vi "Write FIFOs.vi"(7 "Mode":T1, 8 "error in (no error)":errorcluster, 11 "RT Data in":T2 {"Label Transfer Config"."Block Data Refs"."Data Reference" format="%.0x"; "Status Config"."HWOut Dur Ref" format="%.0x"; "Status Config"."HWIn Dur Ref" format="%.0x"; "Status Config"."Error Data Ref" format="%.0x"; "HWOutput Channels"."Labels Settings"."Label" format="%.0o"; "HWInput Channels"."Labels Settings"."Label" format="%.0o"}) -> (0 "error out":errorcluster, 3 "RT Data out":T2 {"Label Transfer Config"."Block Data Refs"."Data Reference" format="%.0x"; "Status Config"."HWOut Dur Ref" format="%.0x"; "Status Config"."HWIn Dur Ref" format="%.0x"; "Status Config"."Error Data Ref" format="%.0x"; "HWOutput Channels"."Labels Settings"."Label" format="%.0o"; "HWInput Channels"."Labels Settings"."Label" format="%.0o"})   [LabVIEW 2017]
uses:
  RT Controls/RT Data.ctl
  RT Controls/RT HW Channel.ctl
  RT Controls/RT Label Settings.ctl
  Shared/Controls and Global/Label.ctl
  Shared/Controls and Global/transferPeriod.ctl
  RT Controls/Driver Data.ctl
  RT Controls/RT Word Settings.ctl
  <vilib>/NI Veristand/Custom Device API/Block Data Reference.ctl
  <vilib>/NI Veristand/Custom Device API/Data Reference.ctl
  RT Controls/RT Param Setting.ctl
  Shared/Controls and Global/Start Bit.ctl
  Shared/Controls and Global/Number of Bits.ctl
  Shared/Controls and Global/TransferType.ctl
  RT Controls/Error Qs.ctl
  RT Controls/Status Channels Config.ctl
  RT Controls/FIFO.ctl
  RT Controls/Label Transfer Config.ctl
  RT Controls/ReadWrite Selector.ctl
  Shared/Ballard Arinc-429 Shared.lvlib
  <vilib>/NI Veristand/Custom Device API/Custom Device API.lvlib
  Ballard Arinc-429 Engine.lvlib
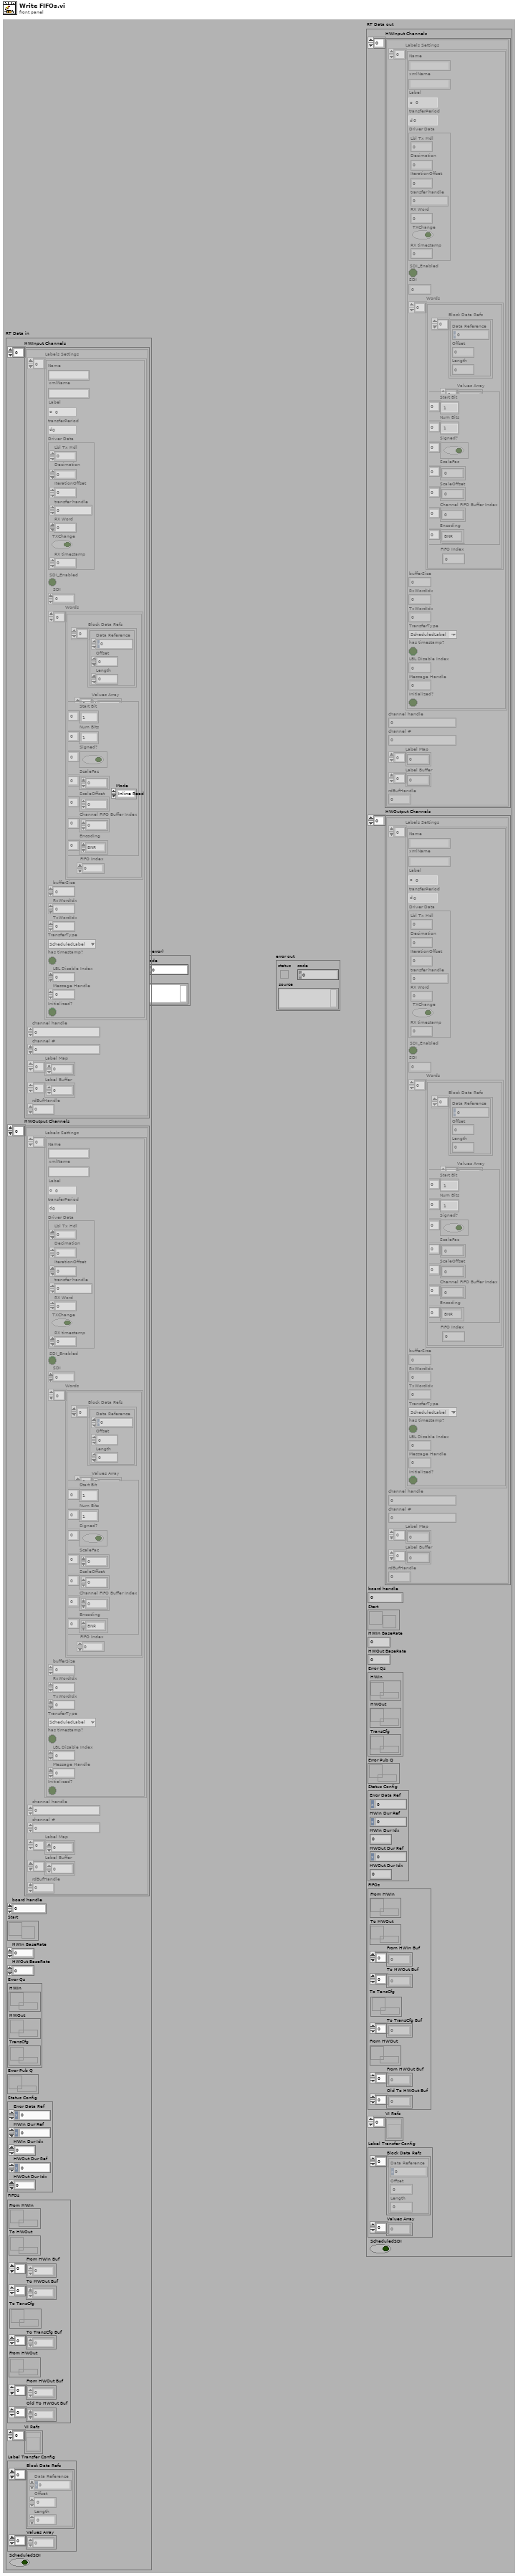
[diagram p1: front panel]
types:
  T1 = typedef "Ballard Arinc-429 Engine.lvlib/ReadWrite Selector.ctl" = enum16{"Inline Read", "Inline Write", "Async HWIn", "Async HWOut"}
  T2 = typedef "Ballard Arinc-429 Engine.lvlib/RT Data.ctl" = cluster{"HWInput Channels":T3[], "HWOutput Channels":T3[], "board handle":u32, "Start":refnum<notifier>, "HWIn BaseRate":i64, "HWOut BaseRate":i64, "Error Qs":T15, "Error Pub Q":refnum<queue>, "Status Config":T16, "FIFOs":T17, "VI Refs":refnum<vi>[], "Label Transfer Config":T18, "ScheduledSDI":bool}
  T3 = typedef "Ballard Arinc-429 Engine.lvlib/RT HW Channel.ctl" = cluster{"Labels Settings":T4[], "channel handle":u32, "channel #":u16, "Label Map":i32[], "Label Buffer":u32[], "rdBufHandle":u32}
  T4 = typedef "Ballard Arinc-429 Engine.lvlib/RT Label Settings.ctl" = cluster{"Name":string, "xmlName":string, "Label":T5, "transferPeriod":T6, "Driver Data":T7, "SDI_Enabled":bool, "SDI":u8, "Words":T8[], "bufferSize":u32, "RxWordIdx":i32, "TxWordIdx":i32, "TransferType":T14, "has timestamp?":bool, "LBL Disable Index":i32, "Message Handle":u64, "Initialized?":bool}
  T5 = typedef "Ballard Arinc-429 Shared.lvlib/Label.ctl" = u8
  T6 = typedef "Ballard Arinc-429 Shared.lvlib/transferPeriod.ctl" = u32
  T7 = typedef "Driver Data.ctl" = cluster{"Lbl Tx Hdl":u32, "Decimation":i32, "IterationOffset":i32, "transfer handle":u32, "RX Word":u32, "TXChange":bool, "RX timestamp":dbl}
  T8 = typedef "Ballard Arinc-429 Engine.lvlib/RT Word Settings.ctl" = cluster{"Block Data Refs":T9[], "Values Array":dbl[], "Length":i32, "FIFO Index":i32, "Param Setting":T11}
  T9 = typedef "Custom Device API.lvlib/Block Data Reference.ctl" = cluster{"Data Reference":T10, "Offset":u64, "Length":u64}
  T10 = typedef "Custom Device API.lvlib/Data Reference.ctl" = i32
  T11 = typedef "Ballard Arinc-429 Engine.lvlib/RT Param Setting.ctl" = cluster{"Start Bit":T12[], "Num Bits":T13[], "Signed?":bool[], "ScaleFac":dbl[], "ScaleOffset":dbl[], "Channel FIFO Buffer Index":i32[], "Encoding":enum16{"BNR", "BCD", "Discrete"}[]}
  T12 = typedef "Ballard Arinc-429 Shared.lvlib/Start Bit.ctl" = i32
  T13 = typedef "Ballard Arinc-429 Shared.lvlib/Number of Bits.ctl" = i32
  T14 = typedef "Ballard Arinc-429 Shared.lvlib/TransferType.ctl" = enum16{"ScheduledLabel", "Acyclic", "Block", "Strobe"}
  T15 = typedef "Error Qs.ctl" = cluster{"HWIn":refnum<queue>, "HWOut":refnum<queue>, "TransCfg":refnum<queue>}
  T16 = typedef "Ballard Arinc-429 Engine.lvlib/Status Channels Config.ctl" = cluster{"Error Data Ref":T10, "HWIn Dur Ref":T10, "HWIn Dur Idx":i32, "HWOut Dur Ref":T10, "HWOut Dur Idx":i32}
  T17 = typedef "FIFO.ctl" = cluster{"From HWIn":refnum<k33>, "To HWOut":refnum<k33>, "From HWIn Buf":dbl[], "To HWOut Buf":dbl[], "To TansCfg":refnum<k33>, "To TransCfg Buf":dbl[], "From HWOut":refnum<k33>, "From HWOut Buf":dbl[], "Old To HWOut Buf":dbl[]}
  T18 = typedef "Ballard Arinc-429 Engine.lvlib/Label Transfer Config.ctl" = cluster{"Block Data Refs":T9[], "Values Array":dbl[]}
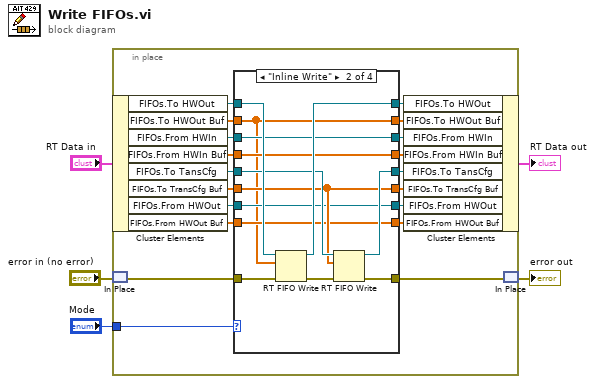
[diagram p0: block diagram]
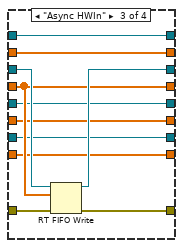
[diagram p3: hidden frame]
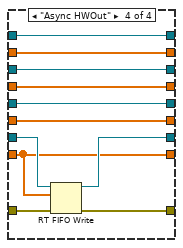
[diagram p4: hidden frame]
diagram:
  n1 = in-place {
    in-place-border: "Mode" -> [w18]
    n2 = in-place-cluster #1("RT Data in") -> ("FIFOs.To HWOut"=w17:refnum<k33>, "FIFOs.To HWOut Buf"=w16:dbl[], "FIFOs.From HWIn"=w24:refnum<k33>, "FIFOs.From HWIn Buf"=w23:dbl[], "FIFOs.To TansCfg"=w13:refnum<k33>, "FIFOs.To TransCfg Buf"=w11:dbl[], "FIFOs.From HWOut"=w9:refnum<k33>, "FIFOs.From HWOut Buf"=w8:dbl[])
    n3 = in-place-match #2("error in (no error)") -> (w20:errorcluster)
    n4 = case shown="\"Inline Write\"" w18 {
      tunnel: w24 -> [w32 w42 w53 w61]
      tunnel: w23 -> [w33 w43 w51 w64]
      tunnel: [w33 w43 w51 w64] -> w22
      tunnel: [w32 w42 w52 w61] -> w21
      tunnel: w20 -> [w31 w46 w57 w68]
      tunnel: [w31 w37 w56 w67] -> w19
      tunnel: w17 -> [w29 w45 w55 w66]
      tunnel: w16 -> [w30 w34 w54 w65]
      tunnel: [w29 w44 w55 w66] -> w15
      tunnel: [w30 w34 w54 w65] -> w14
      tunnel: w13 -> [w28 w41 w50 w63]
      tunnel: [w28 w40 w50 w63] -> w12
      tunnel: w11 -> [w27 w39 w49 w62]
      tunnel: [w27 w39 w49 w62] -> w10
      tunnel: w9 -> [w26 w36 w48 w60]
      tunnel: w8 -> [w25 w35 w47 w58]
      tunnel: [w26 w36 w48 w59] -> w7
      tunnel: [w25 w35 w47 w58] -> w6
      frame Default {
      }
      frame "Inline Write" {
        n5 = RT FIFO Write(0:w45, 1:w34, 3:w46) -> (8:w44:refnum<k33>, 11:w38:errorcluster)  [unwired: 2 in, 2 out]
        n6 = RT FIFO Write(0:w41, 1:w39, 3:w38) -> (8:w40:refnum<k33>, 11:w37:errorcluster)  [unwired: 2 in, 2 out]
      }
      frame "Async HWIn" {
        n7 = RT FIFO Write(0:w53, 1:w51, 3:w57) -> (8:w52:refnum<k33>, 11:w56:errorcluster)  [unwired: 2 in, 2 out]
      }
      frame "Async HWOut" {
        n8 = RT FIFO Write(0:w60, 1:w58, 3:w68) -> (8:w59:refnum<k33>, 11:w67:errorcluster)  [unwired: 2 in, 2 out]
      }
    }
    n9 = in-place-cluster #1("FIFOs.To HWOut"=w15, "FIFOs.To HWOut Buf"=w14, "FIFOs.From HWIn"=w21, "FIFOs.From HWIn Buf"=w22, "FIFOs.To TansCfg"=w12, "FIFOs.To TransCfg Buf"=w10, "FIFOs.From HWOut"=w7, "FIFOs.From HWOut Buf"=w6) -> (→"RT Data out":T2)
    n10 = in-place-match #2(w19) -> (→"error out":errorcluster)
  }
